vi "Datasheet Group Results.vi"(11 "Field Information":T1[](array[typedef])) -> (3 "Each item tests - Grouped Results":cluster{"Result Group":T1[]}[](array[cluster]))   [LabVIEW 2011]
uses:
  www/cgi-bin/_cgi-lib/TDM_INDEX Record.ctl
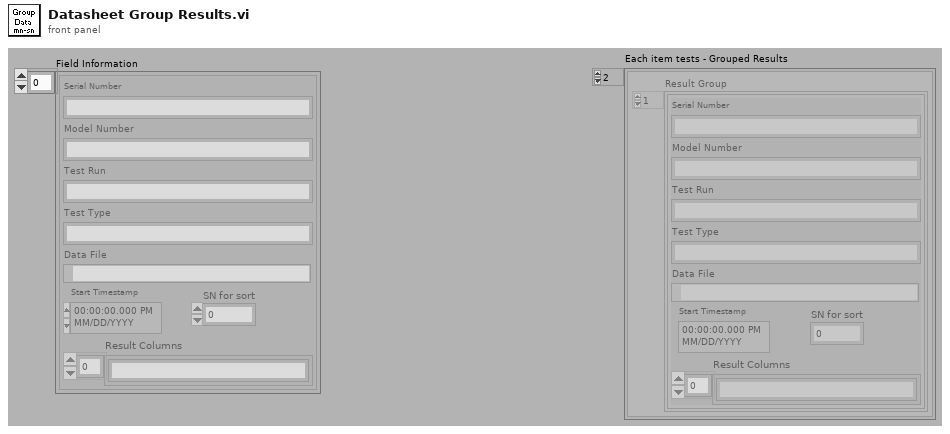
[diagram p1: front panel]
types:
  T1 = typedef "TDM_INDEX Record.ctl" = cluster{"Model Number":string, "SN for sort":i32, "Test Type":string, "Test Run":string, "Serial Number":string, "Start Timestamp":timestamp, "Data File":path, "Result Columns":string[]}
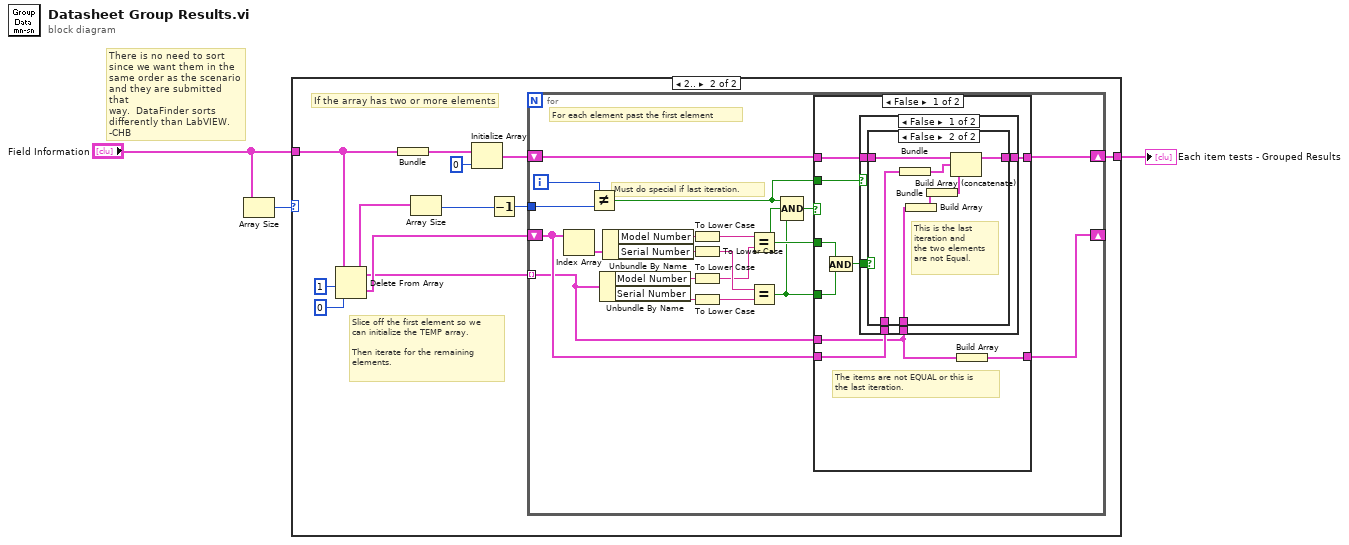
[diagram p0: block diagram]
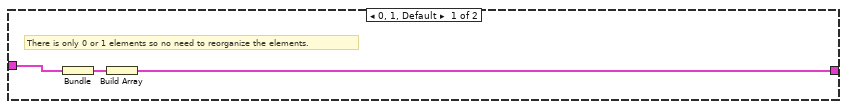
[diagram p2: hidden frame]
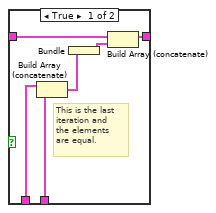
[diagram p3: hidden frame]
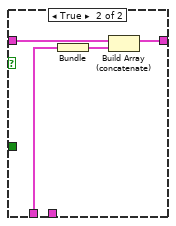
[diagram p4: hidden frame]
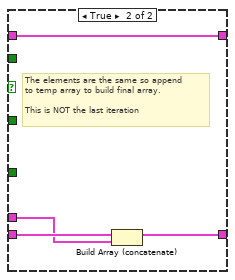
[diagram p5: hidden frame]
diagram:
  # "There is no need to sort\nsince we want them in the\nsame order as the scenario\nand they are submitted that\nway.  DataFinder sorts\ndifferently than LabVIEW.\n-CHB"
  n1 = Array Size(array="Field Information") -> (size(s)=w2:i32)
  n2 = case shown="2.." w2 {
    tunnel: [w4 w15] -> w3
    tunnel: "Field Information" -> [w6 w10]
    frame 0, 1, Default {
      # "There is only 0 or 1 elements so no need to reorganize the elements."
      n3 = Bundle("Field Information"=w6) -> (w5:cluster{"Field Information":T1[]})  [unwired: 1 in]
      n4 = Build Array(w5) -> (w4:cluster{"Field Information":T1[]}[])
    }
    frame 2.. {
      # "Slice off the first element so we\ncan initialize the TEMP array.\n\nThen iterate for the remaining\nelements."
      # "If the array has two or more elements"
      n5 = Delete From Array(array=w10, length=1, index=0 ("dimension size")) -> (deleted portion=w12:T1[], array with subset deleted=w8:T1[])
      n6 = Bundle("Field Information"=w10) -> (w11:cluster{"Field Information":T1[]})  [unwired: 1 in]
      n7 = Array Size(array=w8) -> (size(s)=w7:i32)
      n8 = Initialize Array(w11, 0 ("dimension size")) -> (w16:cluster{"Field Information":T1[]}[])
      n9 = Decrement(x=w7) -> (x-1=w9:i32)
      n10 = for {
        tunnel: w8 -> [w22] mode=indexing
        shift-right: [w32] -> w15
        shift-left: w16 -> [w33]
        shift-right: [w21] -> _
        shift-left: w12 -> [w23]
        tunnel: w9 -> [w26]
        i -> [w25]
        # "For each element past the first element"
        # "Must do special if last iteration."
        n11 = Index Array(array=w23) -> (element=w24:T1)  [unwired: 1 in]
        n12 = Not Equal?(x=w25, y=w26) -> (x != y?=w20:bool)
        n13 = Unbundle By Name(w22) -> ("Model Number"=w36:string, "Serial Number"=w34:string)
        n14 = Unbundle By Name(w24) -> ("Model Number"=w37:string, "Serial Number"=w35:string)
        n15 = To Lower Case(string=w37) -> (all lower case string=w31:string)
        n16 = To Lower Case(string=w35) -> (all lower case string=w30:string)
        n17 = To Lower Case(string=w36) -> (all lower case string=w29:string)
        n18 = To Lower Case(string=w34) -> (all lower case string=w28:string)
        n19 = Equal?(x=w31, y=w29) -> (x = y?=w19:bool)
        n20 = Equal?(x=w30, y=w28) -> (x = y?=w18:bool)
        n21 = Compound Arithmetic op=AND(w20, w19, w18) -> (w27:bool)
        n22 = case shown="False" w27 {
          tunnel: w22 -> [w43 w71]
          tunnel: w23 -> [w44 w72]
          tunnel: [w42 w70] -> w21
          tunnel: w33 -> [w46 w69]
          tunnel: [w45 w69] -> w32
          tunnel: w20 -> [w38 _]
          tunnel: w19 -> [w41 _]
          tunnel: w18 -> [w40 _]
          frame False {
            # "The items are not EQUAL or this is\nthe last iteration."
            n23 = And(x=w41, y=w40) -> (x .and. y?=w39:bool)
            n24 = case shown="False" w38 {
              tunnel: w46 -> [w51 w67]
              tunnel: [w50 w66] -> w45
              tunnel: w44 -> [w49 w65]
              tunnel: w43 -> [w48 _]
              tunnel: w39 -> [w47 _]
              frame False {
                n25 = case shown="False" w47 {
                  tunnel: w51 -> [w57 w64]
                  tunnel: [w56 w63] -> w50
                  tunnel: w49 -> [w54 w62]
                  tunnel: w48 -> [w53 w60]
                  frame True {
                    # "This is the last \niteration and\nthe elements \nare equal."
                    n26 = Build Array (concatenate)(w54, w53) -> (w52:T1[])
                    n27 = Bundle(w52) -> (w55:cluster{T1[]})  [unwired: 1 in]
                    n28 = Build Array (concatenate)(w57, w55) -> (w56:cluster{"Field Information":T1[]}[])
                  }
                  frame False {
                    # "This is the last \niteration and \nthe two elements\nare not Equal."
                    n29 = Bundle("Field Information"=w62) -> (w61:cluster{"Field Information":T1[]})  [unwired: 1 in]
                    n30 = Build Array(w60) -> (w59:T1[])
                    n31 = Bundle(w59) -> (w58:cluster{T1[]})  [unwired: 1 in]
                    n32 = Build Array (concatenate)(w64, w61, w58) -> (w63:cluster{"Field Information":T1[]}[])
                  }
                }
              }
              frame True {
                n33 = Bundle("Field Information"=w65) -> (w68:cluster{"Field Information":T1[]})  [unwired: 1 in]
                n34 = Build Array (concatenate)(w67, w68) -> (w66:cluster{"Field Information":T1[]}[])
              }
            }
            n35 = Build Array(w43) -> (w42:T1[])
          }
          frame True {
            # "The elements are the same so append\nto temp array to build final array.\n\nThis is NOT the last iteration"
            n36 = Build Array (concatenate)(w72, w71) -> (w70:T1[])
          }
        }
      }
    }
  }
  "Each item tests - Grouped Results" <- w3
